vi "Handle Error.vi"(8 "error in":errorcluster, 11 "MSS Target Actor in":refnum<class "MSS Target Actor.lvclass">) -> (0 "error out":errorcluster, 2 "stop actor?":bool=TRUE, 3 "MSS Target Actor out":refnum<class "MSS Target Actor.lvclass">)   [LabVIEW 2023, in "MSS Target Actor.lvlib" / "MSS Target Actor.lvclass"]
doc: "(<B>Filename</B>: Actor Framework.lvlib:Actor.lvclass:Handle Error.vi)\n\nDefines how the actor handles an error that occurred while processing a message. By default, this method does nothing except stop the actor."
uses:
  MSS Target Actor.lvclass
  <vilib>/ActorFramework/Actor/Actor.lvclass
  MSS Target Actor.lvclass/MSS Target Actor.ctl
  Study/Study Actor/IStudy Actor Messages/Log Target Msg/Log Target Msg.lvclass
  <vilib>/Utility/error.llb/DialogType.ctl
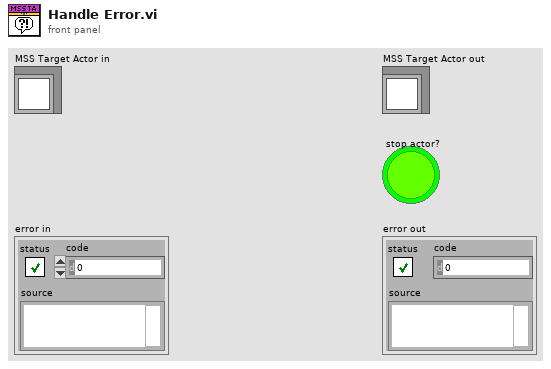
[diagram p1: front panel]
types:
  T1 = typedef "DialogType.ctl" = u16
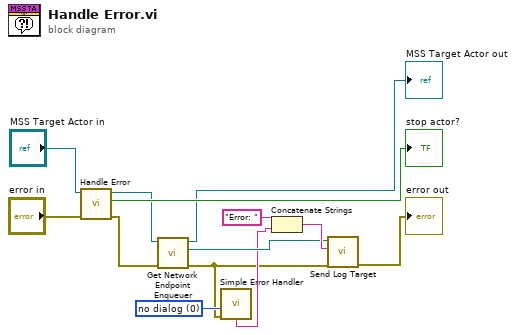
[diagram p0: block diagram]
diagram:
  w3 = T1 0 items=["no dialog", "OK message", "continue or stop message", "OK message + warnings", "continue/stop + warnings"] ("type of dialog (OK msg:1)")
  n1 = call-parent "Handle Error.vi"("error in (no error)"="error in", "Actor in"="MSS Target Actor in") -> ("error out"=w7:errorcluster, "stop actor?"=→"stop actor?":bool, "Actor out"=w5:refnum<class "MSS Target Actor.lvclass">)  [unwired: 7 in]
  n2 = call "Get Network Endpoint Enqueuer.vi"("error in"=w7, "MSS Target Actor in"=w5) -> ("error out"=w1:errorcluster, "Enqueuer"=w8:refnum<class "Message Enqueuer.lvclass">, "MSS Target Actor out"=→"MSS Target Actor out":refnum<class "MSS Target Actor.lvclass">)  [unwired: 7 in]
  n3 = call <vilib>:"Simple Error Handler.vi"("type of dialog (OK msg:1)"=w3, "error in (no error)"=w1) -> ("message"=w2:string)  [unwired: 3 in, 4 out]
  n4 = Concatenate Strings("Error: " ("string"), w2) -> (w9:string)
  n5 = call "Send Log Target.vi"("error in (no error)"=w1, "Entry"=w9, "Message Enqueuer"=w8) -> ("error out"=→"error out":errorcluster)  [unwired: 7 in, 1 out]
